vi "Configure Waveform.vi"(0 "VISA resource name":refnum<visa-resource-name>, 1 "Waveform Name (\"ARB1\")":string="ARB1", 2 "Waveform Type (0:Sinusoid)":u16(ring) items=["Sinusoid", "Square", "Clipped Sinusiod", "User Defined"], 5 "Waveform Mode (0: Fixed)":i32(ring) items=["Fixed", "Step", "Pulse", "List"], 7 "Triggered Waveform Type (0:Sinusoid)":u16(ring) items=["Sinusoid", "Square", "Clipped Sinusiod", "User Defined"], 9 "Triggered Waveform Name (\"ARB1\")":string="ARB1", 11 "error in (no error)":errorcluster, 12 "Waveform Clipping Level (0%)":i32) -> (4 "VISA resource name out":refnum<visa-resource-name>, 15 "error out":errorcluster)   [LabVIEW 2013, in "Cal Inst.lvlib" / "California Instruments iX Series.lvlib"]
doc: "Configures the waveform function of the AC source to output."
uses:
  California Instruments iX Series.lvlib
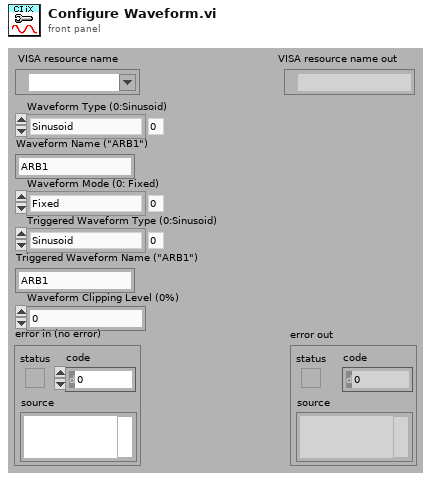
[diagram p1: front panel]
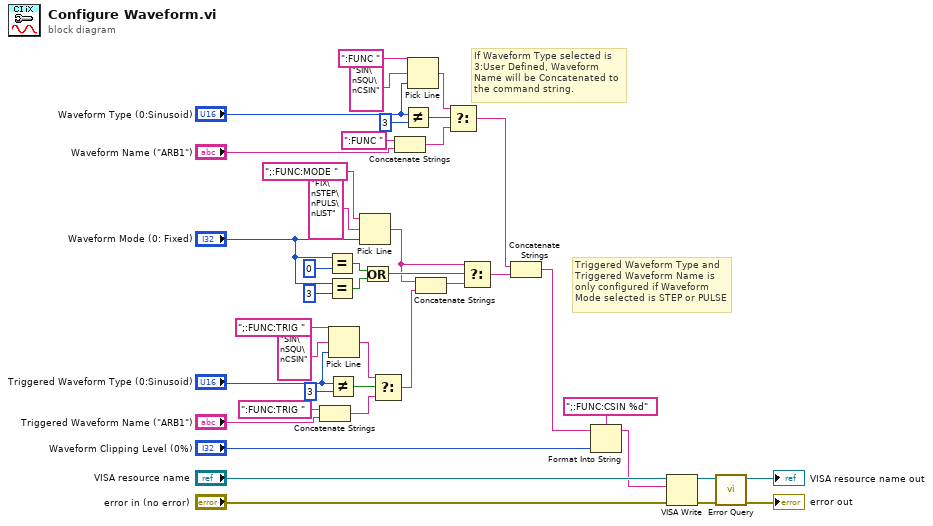
[diagram p0: block diagram]
diagram:
  # "If Waveform Type selected is 3:User Defined, Waveform Name will be Concatenated to the command string."
  # "Triggered Waveform Type and Triggered Waveform Name is only configured if Waveform Mode selected is STEP or PULSE"
  n1 = Concatenate Strings(":FUNC:TRIG " ("string"), "Triggered Waveform Name (\"ARB1\")") -> (w13:string)
  n2 = Equal?(x="Waveform Mode (0: Fixed)", y=0) -> (x = y?=w33:bool)
  n3 = Equal?(x="Waveform Mode (0: Fixed)", y=3) -> (x = y?=w32:bool)
  n4 = Not Equal?(x="Triggered Waveform Type (0:Sinusoid)", y=u16 3) -> (x != y?=w16:bool)
  n5 = Pick Line(string ("")=";:FUNC:TRIG ", multi-line string="SIN\nSQU\nCSIN", line index="Triggered Waveform Type (0:Sinusoid)") -> (output string=w15:string)
  n6 = Pick Line(string ("")=";:FUNC:MODE ", multi-line string="FIX\nSTEP\nPULS\nLIST", line index="Waveform Mode (0: Fixed)") -> (output string=w7:string)
  n7 = Or(x=w33, y=w32) -> (x .or. y?=w10:bool)
  n8 = Select(t=w15, s=w16, f=w13) -> (s? t:f=w9:string)
  n9 = Concatenate Strings(":FUNC " ("string"), "Waveform Name (\"ARB1\")") -> (w24:string)
  n10 = Not Equal?(x="Waveform Type (0:Sinusoid)", y=u16 3) -> (x != y?=w27:bool)
  n11 = Pick Line(string ("")=":FUNC ", multi-line string="SIN\nSQU\nCSIN", line index="Waveform Type (0:Sinusoid)") -> (output string=w26:string)
  n12 = Concatenate Strings(w7, w9) -> (w8:string)
  n13 = Select(t=w26, s=w27, f=w24) -> (s? t:f=w20:string)
  n14 = Select(t=w7, s=w10, f=w8) -> (s? t:f=w6:string)
  n15 = Concatenate Strings(w20, w6) -> (w4:string)
  n16 = Format Into String(format string=";:FUNC:CSIN %d", initial string=w4, "Waveform Clipping Level (0%)") -> (resulting string=w2:string)  [unwired: 1 in, 1 out]
  n17 = VISA Write(VISA resource name="VISA resource name", write buffer=w2, error in (no error)="error in (no error)") -> (VISA resource name out=w39:refnum<visa-resource-name>, error out=w38:errorcluster)  [unwired: 1 out]
  n18 = call "Error Query.vi"("error in (no error)"=w38, "VISA resource name"=w39) -> ("error out"=→"error out":errorcluster, "VISA resource name out"=→"VISA resource name out":refnum<visa-resource-name>)  [unwired: 6 in, 2 out]
